vi "Create Clearpath Nodes.vi"(7 "error in (no error)":errorcluster, 9 "ComHubPortIn":refnum<k24>, 10 "m_SysMgrIn":refnum<k24>) -> (0 "error out":errorcluster, 2 "NodeList":refnum<k24>[](array[refnum]), 3 "m_SysMgrOut":refnum<k24>, 4 "NodeInfo":cluster{"ToString":string, "ToString":string}[](array[cluster]))   [LabVIEW 2020]
uses:
  C:/Users/Jonathan/Documents/Clearpath SDK/CSharp Examples/CLRWrapper/x64/Debug/CLRWrapper.dll
  CSharp Examples/CLRWrapper/x64/Debug/CLRWrapper.dll
panel:
  out "Node Type":T1(ring)
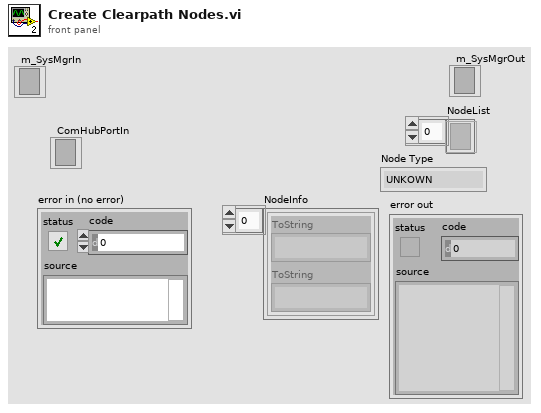
[diagram p1: front panel]
types:
  T1 = enum16{"UNKOWN", "MERIDIAN_ISC", "CLEARPATH_SC", "CLEARPATH_SC_ADV"}
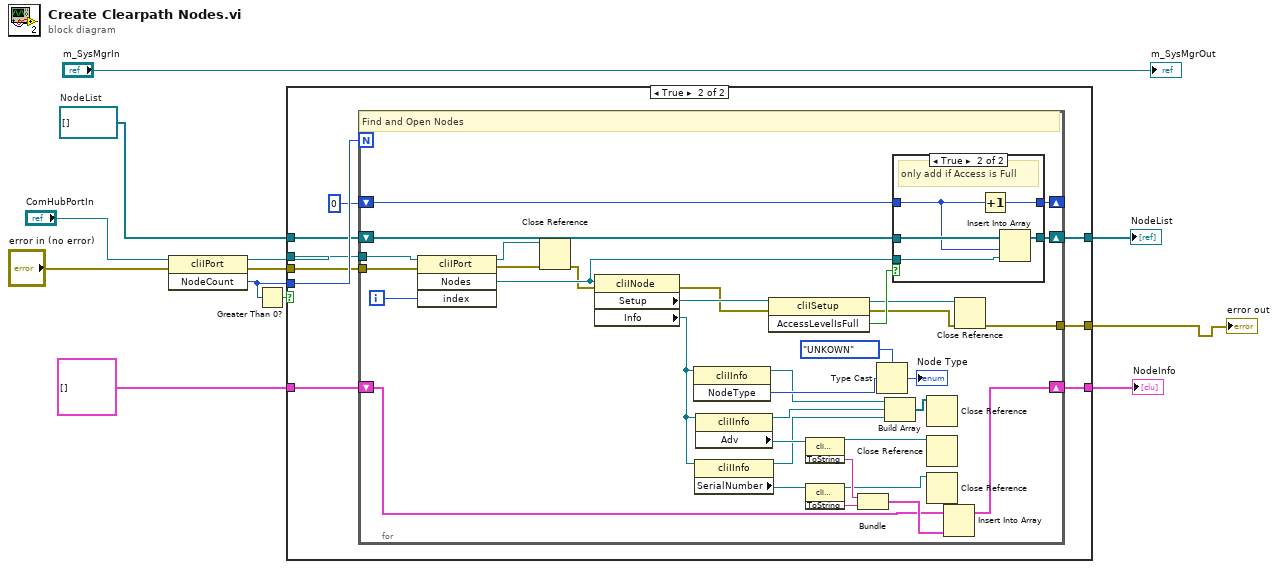
[diagram p0: block diagram]
diagram:
  w3 = refnum<k24>[] []  # NodeList
  n1 = invoke class="cliIPort" method="NodeCount"(reference="ComHubPortIn", error in="error in (no error)") -> (reference out=w8:refnum<k24>, error out=w7:errorcluster, "NodeCount"=w5:u16)  [unwired: 1 in]
  n2 = Greater Than 0?(x=w5) -> (x > 0?=w6:bool)
  n3 = case shown="True" w6 {
    tunnel: w5 -> [_ w23]
    tunnel: w8 -> [_ w22]
    tunnel: w7 -> [w13 w21]
    tunnel: cluster{"ToString":string, "ToString":string}[] [] -> [w14 w20]
    tunnel: [_ w19] -> w11
    tunnel: [w14 w18] -> w12
    tunnel: w3 -> [_ w17]
    tunnel: [w13 w15] -> w2
    frame False {
    }
    frame True {
      n4 = for {
        N: w23 -> [_]
        tunnel: w22 -> [w57]
        tunnel: w21 -> [w56]
        shift-right: [w49] -> w18
        shift-left: w20 -> [w50]
        shift-right: [w46] -> w19
        shift-left: w17 -> [w48]
        shift-right: [w37] -> _
        shift-left: u16 0 ("NodeCount") -> [w38]
        tunnel: [w24] -> w15
        i -> [w47]
        # "Find and Open Nodes"
        n5 = invoke class="cliIPort" method="Nodes"(reference=w57, error in=w56, "index"=w47) -> (reference out=w35:refnum<k24>, error out=w36:errorcluster, "Nodes"=w41:refnum<k24>)  [unwired: 1 in, 1 out]
        n6 = Close Reference(reference=w35, error in (no error)=w36) -> (error out=w34:errorcluster)
        n7 = property class="cliINode"(reference=w41, error in=w34) -> (error out=w39:errorcluster, "Setup"=w42:refnum<k24>, "Info"=w33:refnum<k24>)  [unwired: 1 out]
        n8 = invoke class="cliIInfo" method="NodeType"(reference=w33) -> (reference out=w30:refnum<k24>, "NodeType"=w44:i32)  [unwired: 2 in, 1 out]
        n9 = property class="cliIInfo"(reference=w33) -> (reference out=w32:refnum<k24>, "SerialNumber"=w55:refnum<k24>)  [unwired: 1 in, 1 out]
        n10 = property class="cliIInfo"(reference=w33) -> (reference out=w31:refnum<k24>, "Adv"=w52:refnum<k24>)  [unwired: 1 in, 1 out]
        n11 = invoke class="cliISetup" method="AccessLevelIsFull"(reference=w42, error in=w39) -> (reference out=w26:refnum<k24>, error out=w25:errorcluster, "AccessLevelIsFull"=w40:bool)  [unwired: 1 in]
        n12 = invoke class="cliIInfoAdv" method="ToString"(reference=w52) -> (reference out=w28:refnum<k24>, "ToString"=w51:string)  [unwired: 2 in, 1 out]
        n13 = invoke class="cliValueUnsigned" method="ToString"(reference=w55) -> (reference out=w27:refnum<k24>, "ToString"=w54:string)  [unwired: 2 in, 1 out]
        n14 = Bundle("ToString"=w51, "ToString"=w54) -> (w53:cluster{"ToString":string, "ToString":string})  [unwired: 1 in]
        n15 = Type Cast(type=T1."UNKOWN", x=w44) -> (*(type *) &x=→"Node Type":T1)
        n16 = Build Array(w30, w31, w32) -> (w29:refnum<k24>[])
        n17 = case shown="True" w40 {
          tunnel: w48 -> [w58 w64]
          tunnel: [w58 w63] -> w46
          tunnel: w41 -> [_ w62]
          tunnel: w38 -> [w59 w61]
          tunnel: [w59 w60] -> w37
          frame False {
            # "only add if Access is Full"
          }
          frame True {
            # "only add if Access is Full"
            n18 = Increment(x=w61) -> (x+1=w60:u16)
            n19 = Insert Into Array(array=w64, index=w61, new element=w62) -> (w63:refnum<k24>[])
          }
        }
        n20 = Close Reference(reference=w29) -> ()  [unwired: 1 in, 1 out]
        n21 = Close Reference(reference=w28) -> ()  [unwired: 1 in, 1 out]
        n22 = Close Reference(reference=w27) -> ()  [unwired: 1 in, 1 out]
        n23 = Insert Into Array(array=w50, new element=w53) -> (w49:cluster{"ToString":string, "ToString":string}[])  [unwired: 1 in]
        n24 = Close Reference(reference=w26, error in (no error)=w25) -> (error out=w24:errorcluster)
      }
    }
  }
  "NodeList" <- w11
  "NodeInfo" <- w12
  "error out" <- w2
  "m_SysMgrOut" <- "m_SysMgrIn"
